vi "PS35_Disconnect.vi"(2 "error in (no error)":errorcluster, 3 "Control unit ID":i32=1 min=1 max=10) -> (0 "error out":errorcluster)   [LabVIEW 2020]
doc: "PS35_Disconnect.vi, created: 03.03.2009 alex; last change: 22.10.2019 alex;\n\n<B>FUNCTION:</B> \n\nDisconnect PS 35.\n----------------------------------------------------------------------------------------\n<B>INPUT:</B>\n[I32] <B>Control unit ID:</B> control unit index. (Default=1, Range=1...10) \n[CLU] <B>error in</B>\n----------------------------------------------------------------------------------------\n<B>OUTPUT:</B>\n[CLU] <B>error out</B>\n----------------------------------------------------------------------------------------\n<B>SUB-VIs:</B>\n----------------------------------------------------------------------------------------\n<B>EXT-Calls:</B>\nps35.dll (V2.01)\n----------------------------------------------------------------------------------------"
uses:
  ps35.dll
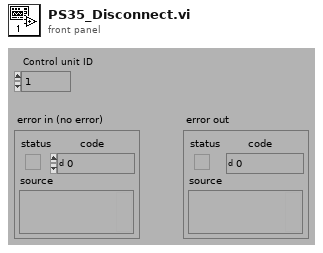
[diagram p1: front panel]
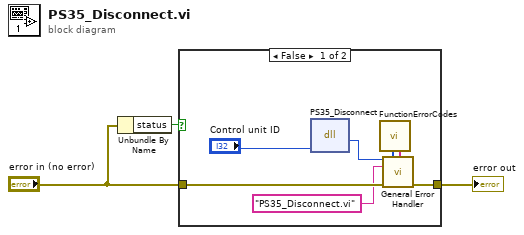
[diagram p0: block diagram]
diagram:
  n1 = Unbundle By Name("error in (no error)") -> ("status"=w1:bool)
  n2 = case shown="False" w1 {
    tunnel: "error in (no error)" -> [w9 w11]
    tunnel: [w8 w11] -> w3
    frame False {
      n3 = dll-call lib="C:/GEECS/Developers Version/source/Device Drivers/OwiSoft_PS35/OWISoftOEM/ps35/labview/lv82/ps35.dll" fn="PS35_Disconnect"("Index"="Control unit ID") -> ("Rückgabetyp"=w7:i32)  [unwired: 4 in, 2 out]
      n4 = call "FunctionErrorCodes.vi"() -> ("[user-defined codes]"=w4:i32[], "[user-defined descriptions]"=w5:string[])  [unwired: 8 in]
      n5 = call "General Error Handler.vi"("[error code] (0)"=w7, "[user-defined codes]"=w4, "[user-defined descriptions]"=w5, "[error source] (\" \")"="PS35_Disconnect.vi" ("[error source] (\" \")"), "error in (no error)"=w9) -> ("error out"=w8:errorcluster)  [unwired: 6 in, 4 out]
    }
    frame True {
    }
  }
  "error out" <- w3
